vi "Hide Key Focus Border.vi"() -> ()   [LabVIEW 2020]
panel:
  in  "stop":bool
  in  "Give Darren's Focus":bool
  in  "Give Standard Focus":bool
  in  "Standard Combo Box":string(combo)
  in  "Darren's Combo Box":string(combo)
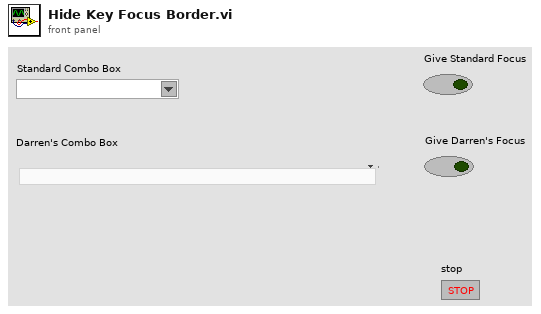
[diagram p1: front panel]
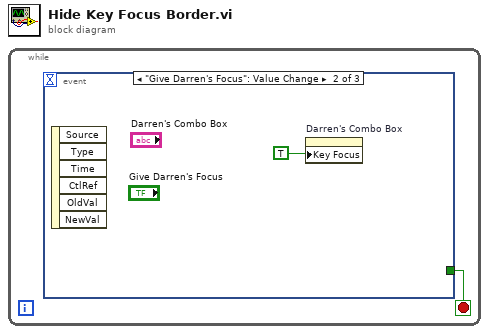
[diagram p0: block diagram]
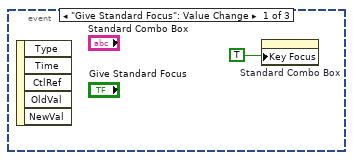
[diagram p2: hidden frame]
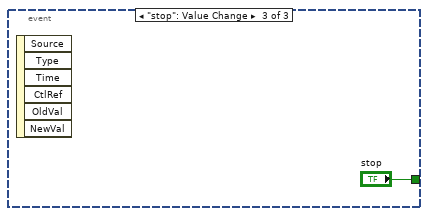
[diagram p3: hidden frame]
diagram:
  n1 = while {
    stop <- w1 stop-if-true
    n2 = event shown="[1] \"Give Darren's Focus\": Value Change" {
      selector: _ -> [_ _ _]
      dyn-events: _ -> [_ _ _]
      timeout: _ -> [_ _ _]
      tunnel: [_ _ "stop"] -> w1
      event "Give Standard Focus": Value Change {
        n3 = event-data() -> ()  [unwired: 1 in, 5 out]
        n4 = property on="Standard Combo Box" class="CmbBox"("Key Focus"=TRUE) -> ()  [unwired: 2 in, 2 out]
      }
      event "Give Darren's Focus": Value Change {
        n5 = event-data() -> ()  [unwired: 1 in, 6 out]
        n6 = property on="Darren's Combo Box" class="CmbBox"("Key Focus"=TRUE) -> ()  [unwired: 2 in, 2 out]
      }
      event "stop": Value Change {
        n7 = event-data() -> ()  [unwired: 1 in, 6 out]
      }
    }
  }
